vi "n2v (SubVI).vi"(9 "Übersetzung ermitteln aus":T1(ring), 10 "Array (Eingang)":dbl[](array[numeric]), 11 "Rollenumfang [m]":dbl) -> (2 "Array (Ausgang)":dbl[](array[numeric]), 3 "Boolesch":bool)   [LabVIEW 2014]
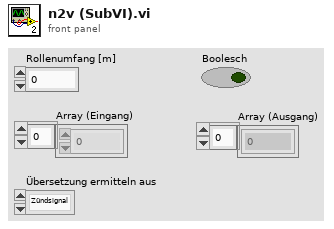
[diagram p1: front panel]
types:
  T1 = enum8{"Zündsignal", "Getriebe & Reifen", "nKuWe / nRolle", "Vario (km/h)"}
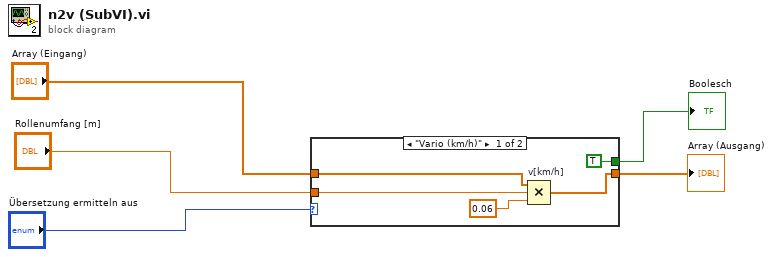
[diagram p0: block diagram]
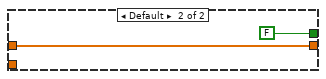
[diagram p2: hidden frame]
diagram:
  n1 = case shown="\"Vario (km/h)\"" "Übersetzung ermitteln aus" {
    tunnel: "Array (Eingang)" -> [w7 w12]
    tunnel: [w9 w12] -> w2
    tunnel: [TRUE FALSE] -> w3
    tunnel: "Rollenumfang [m]" -> [w6 _]
    frame "Vario (km/h)" {
      n2 = Compound Arithmetic op=MULTIPLY "v[km/h]"(w7, w6, 0.06) -> (w9:dbl[])
    }
    frame Default {
    }
  }
  "Boolesch" <- w3
  "Array (Ausgang)" <- w2
